vi "Get Cell View.vi"(11 "Cell View in":refnum<class "Cell View.lvclass">) -> (2 "Cell View":refnum<k24>, 3 "Cell View out":refnum<class "Cell View.lvclass">)   [LabVIEW 2024, in "Cell View.lvclass"]
uses:
  Cell View.lvclass
  D:/git/Sourcegrid-LabVIEW/dll/SourceGrid.dll
  dll/SourceGrid.dll
  Cell View.lvclass/Cell View.ctl
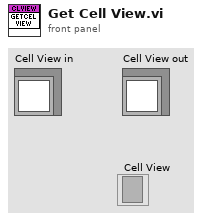
[diagram p1: front panel]
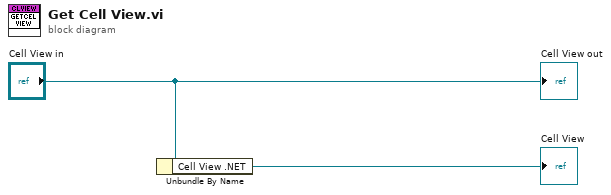
[diagram p0: block diagram]
diagram:
  n1 = Unbundle By Name("Cell View in") -> ("Cell View .NET"=→"Cell View":refnum<k24>)
  "Cell View out" <- "Cell View in"
